vi "Set SCADA stop notifier.vi"(10 "SCADA stop":refnum<notifier>, 11 "SCADA in":refnum<class "SCADA.lvclass">) -> (3 "SCADA out":refnum<class "SCADA.lvclass">)   [LabVIEW 2015, in "SCADA Core.lvlib" / "SCADA.lvclass"]
uses:
  SCADA.lvclass
  SCADA.lvclass/SCADA.ctl
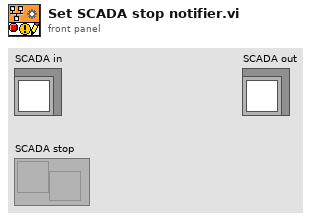
[diagram p1: front panel]
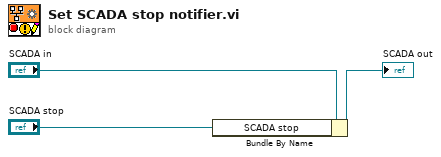
[diagram p0: block diagram]
diagram:
  n1 = Bundle By Name(cluster="SCADA in", "SCADA stop"="SCADA stop") -> (→"SCADA out":refnum<class "SCADA.lvclass">)
